vi "tool_Unicode_Trim Whitespace.vi"(5 "Remove (leading and trailing)":enum16{"leading", "trailing", "both"}(ring)=enum."both", 6 "String in *UTF-16":string) -> (1 "String out *UTF-16":string)   [LabVIEW 2013, in "SET_Unicode Tools.lvlib"]
doc: "Removes leading and/or trailing whitespace from a string.\nWhitespace is defined as any of the following characters (where values are in the format: dec, hex, string):\n <b>tab</b> = 9, 0x09, \\t\n <b>newline</b> = 10, 0x0A, \\n\n <b>vertical tab</b> = 11, 0x0B, \\0B\n <b>form feed</b> = 12, 0x0C, \\f\n <b>carriage return</b> = 13, 0x0D, \\r \n <b>space</b> = 32, 0x20, \\s\n\nThis VI 's execution is set to <b>subroutine</b>\nThis VI is <b>reentrant</b>"
uses:
  SET_Unicode Tools.lvlib
panel:
  # "!!!Modified for Unicode Support!!!"
  # "Trim Whitespace (String) 1.vi\n\nRemoves leading and/or trailing whitespace from a string.\n\nPlease visit http://www.OpenG.org to learn about the\nOpen Source LabVIEW software movement.\n\nNOTICE -- YOU MUST LEAVE THIS NOTICE IN PLACE.  PER THE TERMS OF THE LICENSE BELOW, YOU MAY SUBLICENSE THIS SOFTWARE \nIN ANY WAY THAT DOES NOT CONFLICT WITH THIS LICENSE.\n\n### BSD License (http://www.opensource.org/licenses/bsd-license.php) Begin ###\n\nCopyright (c) 2002-2006, Jim Kring <jim@jimkring.com>\nCopyright (c) 2002, Cal-Bay Systems, Inc. <info@calbay.com>\nCopyright (c) 2011,  Shaun Rumbell <shaunr@labview-tools.com> \nCopyright (c) 2011,  Darin.K <darin@alum.mit.edu>\nCopyright (c) 2011, Jonathon Green <jg@jgcode.net>\n\nAll rights reserved.\n\nRedistribution and use in source and binary forms, with or without modification, are permitted provided that the following conditions are met:\n\n    * Redistributions of source code must retain the above copyright notice, this list of conditions and the following disclaimer.\n    * Redistributions in binary form must reproduce the above copyright notice, this list of conditions and the following disclaimer in the \n       documentation and/or other materials provided with the distribution.\n    * Neither the name of SciWare, James Kring, Inc., nor the names of its contributors may be used to endorse or promote products derived \n       from this software without specific prior written permission.\n\nTHIS SOFTWARE IS PROVIDED BY THE COPYRIGHT HOLDERS AND CONTRIBUTORS \"AS IS\" AND ANY EXPRESS OR IMPLIED WARRANTIES, \nINCLUDING, BUT NOT LIMITED TO, THE IMPLIED WARRANTIES OF MERCHANTABILITY AND FITNESS FOR A PARTICULAR PURPOSE ARE \nDISCLAIMED. IN NO EVENT SHALL THE COPYRIGHT OWNER OR CONTRIBUTORS BE LIABLE FOR ANY DIRECT, INDIRECT, INCIDENTAL,\n SPECIAL, EXEMPLARY, OR CONSEQUENTIAL DAMAGES (INCLUDING, BUT NOT LIMITED TO, PROCUREMENT OF SUBSTITUTE GOODS OR \nSERVICES; LOSS OF USE, DATA, OR PROFITS; OR BUSINESS INTERRUPTION) HOWEVER CAUSED AND ON ANY THEORY OF LIABILITY, \nWHETHER IN CONTRACT, STRICT LIABILITY, OR TORT (INCLUDING NEGLIGENCE OR OTHERWISE) ARISING IN ANY WAY OUT OF THE USE \nOF THIS SOFTWARE, EVEN IF ADVISED OF THE POSSIBILITY OF SUCH DAMAGE.\n\n### BSD License End ###"
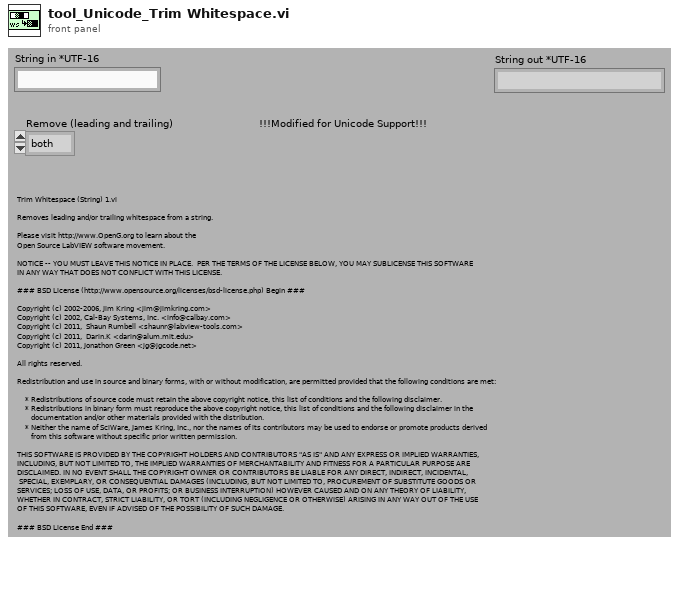
[diagram p1: front panel]
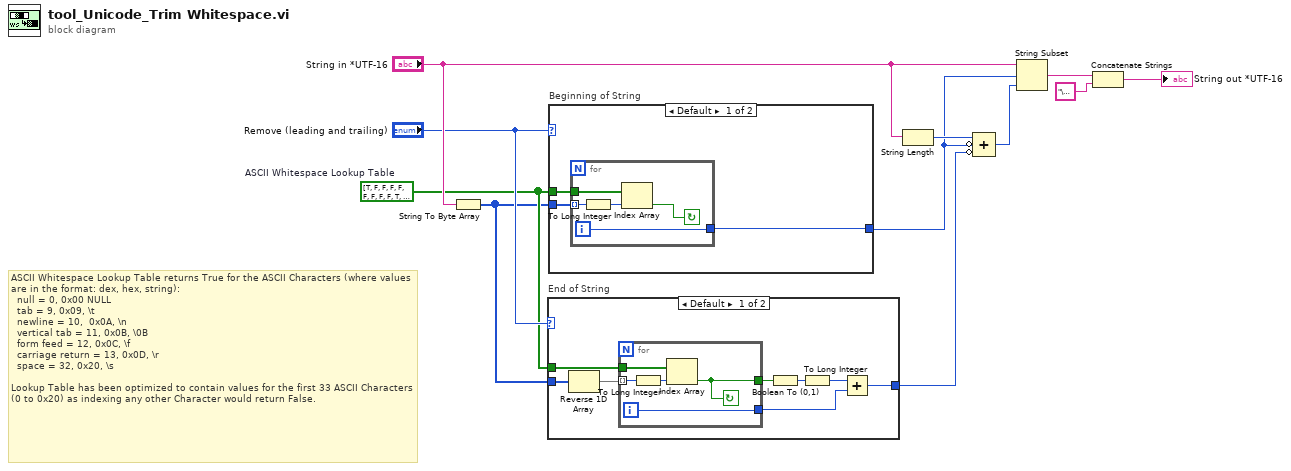
[diagram p0: block diagram]
diagram:
  w5 = bool[] [TRUE, FALSE, FALSE, FALSE, FALSE, FALSE, FALSE, FALSE, FALSE, TRUE, TRUE, TRUE, TRUE, TRUE, FALSE, FALSE, FALSE, FALSE, FALSE, FALSE, FALSE, FALSE, FALSE, FALSE, FALSE, FALSE, FALSE, FALSE, FALSE, FALSE, FALSE, FALSE, TRUE]  # ASCII Whitespace Lookup Table
  # "ASCII Whitespace Lookup Table returns True for the ASCII Characters (where values are in the format: dex, hex, string):\n  null = 0, 0x00 NULL\n  tab = 9, 0x09, \\t\n  newline = 10,  0x0A, \\n\n  vertical tab = 11, 0x0B, \\0B\n  form feed = 12, 0x0C, \\f\n  carriage return = 13, 0x0D, \\r \n  space = 32, 0x20, \\s\n\nLookup Table has been optimized to contain values for the first 33 ASCII Characters (0 to 0x20) as indexing any other Character would return False."
  n1 = String To Byte Array(string="String in *UTF-16") -> (unsigned byte array=w4:u8[])
  n2 = case "End of String" shown="Default" "Remove (leading and trailing)" {
    tunnel: [w18 _] -> w6
    tunnel: w5 -> [w15 _]
    tunnel: w4 -> [w13 _]
    frame Default {
      n3 = Reverse 1D Array(array=w13) -> (reversed array=w12:u8[])
      n4 = for {
        tunnel: w12 -> [w21] mode=indexing
        tunnel: [w24] -> w19
        tunnel: [w22] -> w14
        tunnel: w15 -> [w23]
        i -> [w24]
        stop <- w22 continue-if-true
        n5 = To Long Integer(number=w21) -> (32bit integer=w20:i32)
        n6 = Index Array(array=w23, index=w20) -> (element=w22:bool)
      }
      n7 = Boolean To (0,1)(Boolean=w14) -> (0, 1=w17:i16)
      n8 = To Long Integer(number=w17) -> (32bit integer=w16:i32)
      n9 = Add(x=w16, y=w19) -> (x+y=w18:i32)
    }
    frame "leading" {
    }
  }
  n10 = case "Beginning of String" shown="Default" "Remove (leading and trailing)" {
    tunnel: w4 -> [w27 _]
    tunnel: [w26 _] -> w7
    tunnel: w5 -> [w25 _]
    frame Default {
      n11 = for {
        tunnel: w27 -> [w29] mode=indexing
        tunnel: [w32] -> w26
        tunnel: w25 -> [w31]
        i -> [w32]
        stop <- w30 continue-if-true
        n12 = To Long Integer(number=w29) -> (32bit integer=w28:i32)
        n13 = Index Array(array=w31, index=w28) -> (element=w30:bool)
      }
    }
    frame "trailing" {
    }
  }
  n14 = String Length(string="String in *UTF-16") -> (length=w10:i32)
  n15 = Compound Arithmetic op=ADD(w10, invert w7, invert w6) -> (w11:i32)
  n16 = String Subset(string="String in *UTF-16", offset (0)=w7, length (rest)=w11) -> (substring=w3:string)
  n17 = Concatenate Strings(w3, "\u0000" ("string")) -> (→"String out *UTF-16":string)
